vi "ExpandArray.vi"(11 "Array In":dbl[](array[numeric])) -> (3 "Expanded Array":dbl[](array[numeric]))   [LabVIEW 2024]
uses:
  GlobalVariables.vi
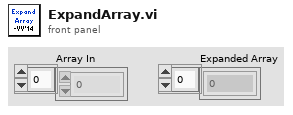
[diagram p1: front panel]
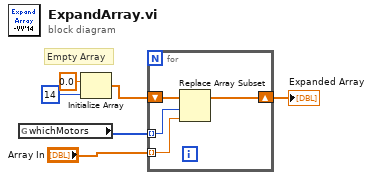
[diagram p0: block diagram]
diagram:
  # "Empty Array"
  n1 = global read "GlobalVariables.vi" "whichMotors"() -> (w1:i32[])
  n2 = Initialize Array(0.0 ("element"), 14 ("dimension size")) -> (w2:dbl[])
  n3 = for {
    tunnel: w1 -> [w10] mode=indexing
    tunnel: "Array In" -> [w7] mode=indexing
    shift-right: [w9] -> w6
    shift-left: w2 -> [w8]
    n4 = Replace Array Subset(array=w8, new element=w7, index=w10) -> (w9:dbl[])
  }
  "Expanded Array" <- w6
